vi "S2C_Shared_Proc_Respond.vi"(8 "Error In":errorcluster, 10 "Settings":T1, 11 "Response":variant) -> (0 "Error Out":errorcluster)   [LabVIEW 2024]
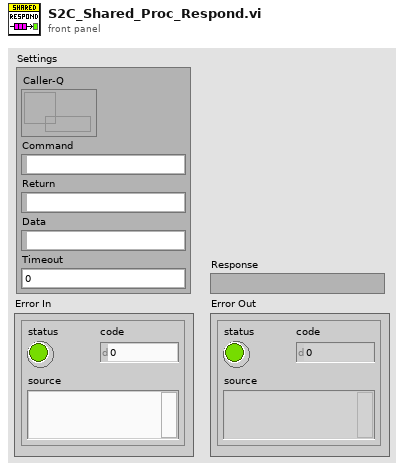
[diagram p1: front panel]
types:
  T1 = cluster{"Caller-Q":refnum<queue>, "Command":string, "Return":string, "Data":variant, "Timeout":dbl}
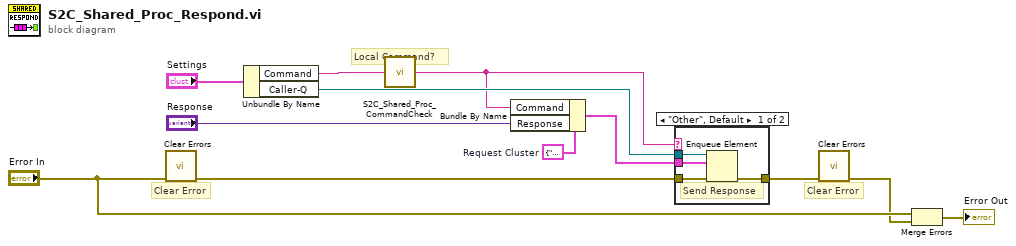
[diagram p0: block diagram]
diagram:
  w11 = cluster{"Command":string, "Response":variant} {"Command"="", "Response"=variant}  # Request Cluster
  # "Clear Error"
  # "Local Command?"
  # "Clear Error"
  n1 = call <vilib>:"Clear Errors.vi"("error in (no error)"="Error In") -> ("error out"=w12:errorcluster)  [unwired: 5 in, 1 out]
  n2 = Unbundle By Name("Settings") -> ("Command"=w2:string, "Caller-Q"=w9:refnum<queue>)
  n3 = call "S2C_Shared_Proc_CommandCheck.vi"("Cmd In"=w2) -> ("Cmd Out"=w1:string)  [unwired: 13 in, 1 out]
  n4 = Bundle By Name(cluster=w11, "Command"=w1, "Response"="Response") -> (w10:cluster{"Command":string, "Response":variant})
  n5 = case shown="\"Other\", Default" w1 {
    tunnel: w9 -> [w16 _]
    tunnel: w12 -> [w15 w17]
    tunnel: [w14 w17] -> w6
    tunnel: w10 -> [w13 _]
    frame "Other", Default {
      # "Send Response"
      n6 = Enqueue Element(queue=w16, element=w13, error in (no error)=w15) -> (error out=w14:errorcluster)  [unwired: 1 in, 2 out]
    }
    frame "Exit", "Init", "None" {
      # "No Response\nCase"
    }
  }
  n7 = call <vilib>:"Clear Errors.vi"("error in (no error)"=w6) -> ("error out"=w4:errorcluster)  [unwired: 5 in, 1 out]
  n8 = Merge Errors("Error In", w4) -> (→"Error Out":errorcluster)
